vi "Prepare Load.vi"(0 "instrument handle":refnum<k15>, 5 "Load Current Level (A)":dbl, 7 "Load Output Function":T1, 11 "error in (no error)":errorcluster) -> (15 "error out":errorcluster)   [LabVIEW 2020]
uses:
  Load Output Function.ctl
  <instrlib>/niDCPower/nidcpower.llb/niDCPower Source Mode.ctl
  <instrlib>/niDCPower/nidcpower.llb/niDCPower Output Function.ctl
  <instrlib>/niDCPower/nidcpower.llb/niDCPower Wait For Event - Event.ctl
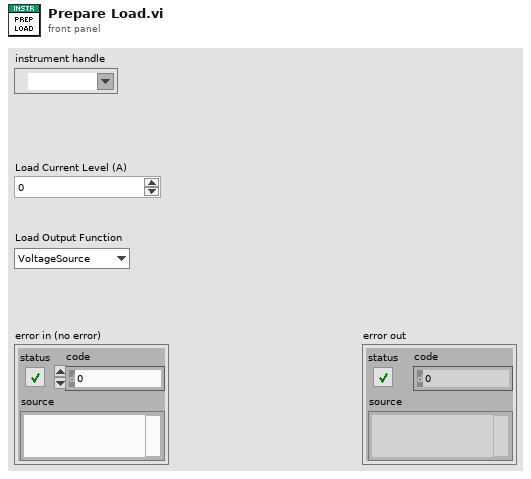
[diagram p1: front panel]
types:
  T1 = typedef "Load Output Function.ctl" = enum16{"VoltageSource", "CurrentSource"}
  T2 = typedef "niDCPower Wait For Event - Event.ctl" = i32
  T3 = typedef "niDCPower Output Function.ctl" = i32
  T4 = typedef "niDCPower Source Mode.ctl" = i32
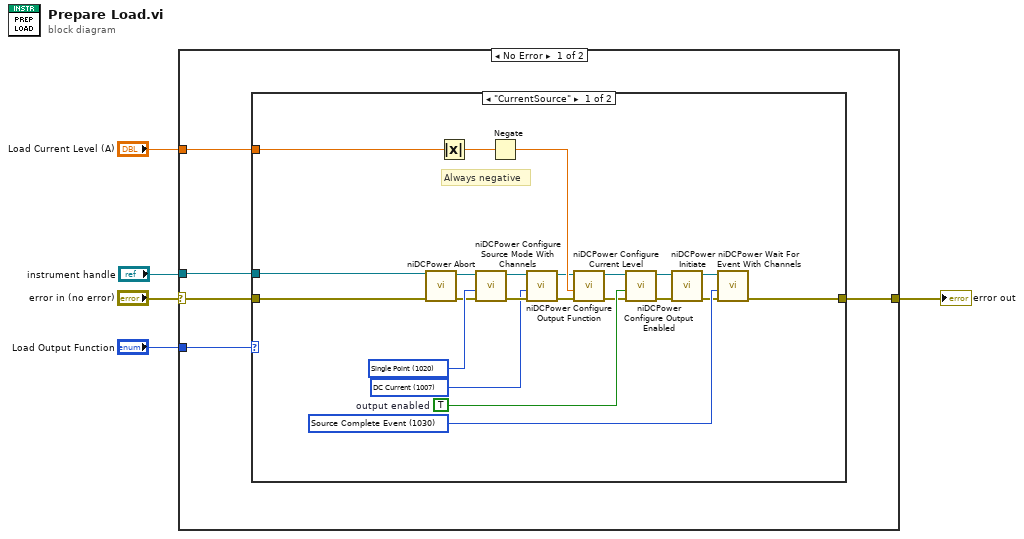
[diagram p0: block diagram]
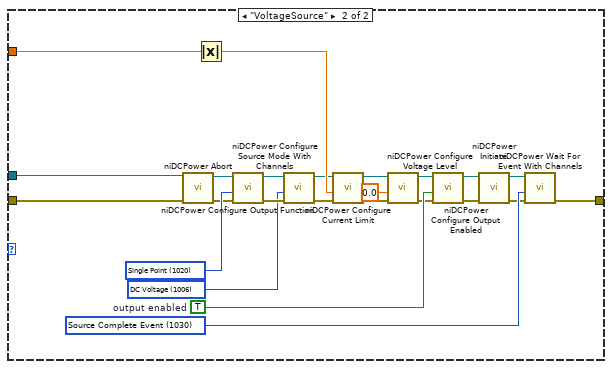
[diagram p2: hidden frame]
diagram:
  n1 = case shown="No Error" "error in (no error)" {
    selector: "error in (no error)" -> [w8 w57]
    tunnel: "Load Current Level (A)" -> [w10 _]
    tunnel: [w9 w57] -> w4
    tunnel: "Load Output Function" -> [w7 _]
    tunnel: "instrument handle" -> [w6 _]
    frame No Error {
      n2 = case shown="\"CurrentSource\"" w7 {
        tunnel: w10 -> [w29 w55]
        tunnel: [w28 w54] -> w9
        tunnel: w8 -> [w25 w33]
        tunnel: w6 -> [w11 w34]
        frame "CurrentSource" {
          w32 = T2 1030 items=["Source Complete Event"=1030, "Measure Complete Event"=1031, "Sequence Iteration Complete Event"=1032, "Sequence Engine Done Event"=1033, "Pulse Complete Event"=1051, "Ready For Pulse Trigger Event"=1052] ("event")
          w22 = TRUE  # output enabled
          w16 = T3 1007 items=["DC Voltage"=1006, "DC Current"=1007, "Pulse Voltage"=1049, "Pulse Current"=1050] ("output function")
          w19 = T4 1020 items=["Single Point"=1020, "Sequence"=1021] ("source mode")
          # "Always negative"
          n3 = call <instrlib>:"niDCPower Abort.vi"("error in (no error)"=w25, "instrument handle"=w11) -> ("error out"=w15:errorcluster, "instrument handle out"=w14:refnum<k15>)  [unwired: 8 in]
          n4 = Absolute Value(x=w29) -> (abs(x)=w30:dbl)
          n5 = call <instrlib>:"niDCPower Configure Source Mode With Channels.vi"("error in (no error)"=w15, "source mode"=w19, "instrument handle"=w14) -> ("error out"=w17:errorcluster, "instrument handle out"=w18:refnum<k15>)  [unwired: 7 in]
          n6 = Negate(x=w30) -> (-x=w31:dbl)
          n7 = call <instrlib>:"niDCPower Configure Output Function.vi"("error in (no error)"=w17, "output function"=w16, "instrument handle"=w18) -> ("error out"=w20:errorcluster, "instrument handle out"=w21:refnum<k15>)  [unwired: 7 in]
          n8 = call <instrlib>:"niDCPower Configure Current Level.vi"("error in (no error)"=w20, "current level"=w31, "instrument handle"=w21) -> ("error out"=w12:errorcluster, "instrument handle out"=w13:refnum<k15>)  [unwired: 7 in]
          n9 = call <instrlib>:"niDCPower Configure Output Enabled.vi"("error in (no error)"=w12, "output enabled"=w22, "instrument handle"=w13) -> ("error out"=w23:errorcluster, "instrument handle out"=w24:refnum<k15>)  [unwired: 7 in]
          n10 = call <instrlib>:"niDCPower Initiate.vi"("error in (no error)"=w23, "instrument handle"=w24) -> ("error out"=w27:errorcluster, "instrument handle out"=w26:refnum<k15>)  [unwired: 8 in]
          n11 = call <instrlib>:"niDCPower Wait For Event With Channels.vi"("error in (no error)"=w27, "event"=w32, "instrument handle"=w26) -> ("error out"=w28:errorcluster)  [unwired: 7 in, 1 out]
        }
        frame "VoltageSource" {
          w56 = T2 1030 items=["Source Complete Event"=1030, "Measure Complete Event"=1031, "Sequence Iteration Complete Event"=1032, "Sequence Engine Done Event"=1033, "Pulse Complete Event"=1051, "Ready For Pulse Trigger Event"=1052] ("event")
          w49 = TRUE  # output enabled
          w45 = T3 1006 items=["DC Voltage"=1006, "DC Current"=1007, "Pulse Voltage"=1049, "Pulse Current"=1050] ("output function")
          w48 = T4 1020 items=["Single Point"=1020, "Sequence"=1021] ("source mode")
          n12 = call <instrlib>:"niDCPower Abort.vi"("error in (no error)"=w33, "instrument handle"=w34) -> ("error out"=w44:errorcluster, "instrument handle out"=w43:refnum<k15>)  [unwired: 8 in]
          n13 = Absolute Value(x=w55) -> (abs(x)=w42:dbl)
          n14 = call <instrlib>:"niDCPower Configure Source Mode With Channels.vi"("error in (no error)"=w44, "source mode"=w48, "instrument handle"=w43) -> ("error out"=w46:errorcluster, "instrument handle out"=w47:refnum<k15>)  [unwired: 7 in]
          n15 = call <instrlib>:"niDCPower Configure Output Function.vi"("error in (no error)"=w46, "output function"=w45, "instrument handle"=w47) -> ("error out"=w41:errorcluster, "instrument handle out"=w40:refnum<k15>)  [unwired: 7 in]
          n16 = call <instrlib>:"niDCPower Configure Current Limit.vi"("error in (no error)"=w41, "current limit"=w42, "instrument handle"=w40) -> ("error out"=w39:errorcluster, "instrument handle out"=w37:refnum<k15>)  [unwired: 7 in]
          n17 = call <instrlib>:"niDCPower Configure Voltage Level.vi"("error in (no error)"=w39, "voltage level"=0.0, "instrument handle"=w37) -> ("error out"=w38:errorcluster, "instrument handle out"=w36:refnum<k15>)  [unwired: 7 in]
          n18 = call <instrlib>:"niDCPower Configure Output Enabled.vi"("error in (no error)"=w38, "output enabled"=w49, "instrument handle"=w36) -> ("error out"=w50:errorcluster, "instrument handle out"=w51:refnum<k15>)  [unwired: 7 in]
          n19 = call <instrlib>:"niDCPower Initiate.vi"("error in (no error)"=w50, "instrument handle"=w51) -> ("error out"=w53:errorcluster, "instrument handle out"=w52:refnum<k15>)  [unwired: 8 in]
          n20 = call <instrlib>:"niDCPower Wait For Event With Channels.vi"("error in (no error)"=w53, "event"=w56, "instrument handle"=w52) -> ("error out"=w54:errorcluster)  [unwired: 7 in, 1 out]
        }
      }
    }
    frame Error {
    }
  }
  "error out" <- w4
